vi "Test11ACiR.vi"(8 "errin":errorcluster, 9 "L2T 2":T1 caption="Limites de test pris en compte", 10 "result string":string, 11 "SN":string) -> (0 "error out":errorcluster, 4 "String":string)   [LabVIEW 2020]
uses:
  Ctrl/L2T.ctl
  <vilib>/regexp/Match Regular Expression.xnode
panel:
  # "Pre DCIR_____________________________________"
  # "intra DCIR_____________________________________"
  # "Post DCIR_____________________________________"
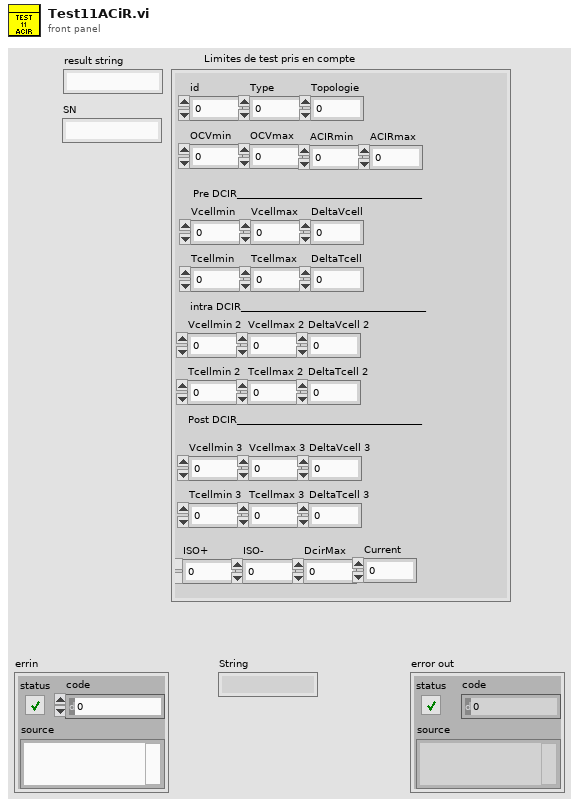
[diagram p1: front panel]
types:
  T1 = typedef "L2T.ctl" = cluster{"id":dbl, "Type":dbl, "OCVmin":dbl, "OCVmax":dbl, "ACIRmin":dbl, "ACIRmax":dbl, "Vcellmin":dbl, "Vcellmax":dbl, "DeltaVcell":dbl, "Tcellmin":dbl, "Tcellmax":dbl, "DeltaTcell":dbl, "ISO+":dbl, "ISO-":dbl, "DcirMax":dbl, "Current":dbl, "Topologie":dbl, "Vcellmin 2":dbl, "Vcellmax 2":dbl, "DeltaVcell 2":dbl, "Tcellmin 2":dbl, "Tcellmax 2":dbl, "DeltaTcell 2":dbl, "Vcellmin 3":dbl, "Vcellmax 3":dbl, "DeltaVcell 3":dbl, "Tcellmin 3":dbl, "Tcellmax 3":dbl, "DeltaTcell 3":dbl}
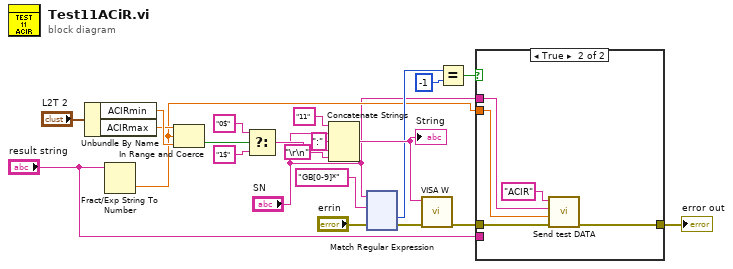
[diagram p0: block diagram]
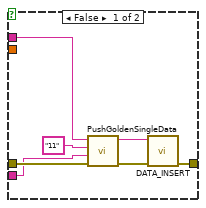
[diagram p2: hidden frame]
diagram:
  n1 = Unbundle By Name("L2T 2") -> ("ACIRmin"=w19:dbl, "ACIRmax"=w18:dbl)
  n2 = Fract/Exp String To Number(string="result string") -> (number=w5:dbl)  [unwired: 3 in, 1 out]
  n3 = In Range and Coerce(upper limit=w18, x=w5, lower limit=w19) -> (In Range?=w20:bool)  [unwired: 1 out]
  n4 = Select(t="0$" ("chaîne"), s=w20, f="1$" ("chaîne")) -> (s? t:f=w17:string)
  n5 = Concatenate Strings("11" ("chaîne"), "SN", ":" ("string"), w17, "\r\n") -> (w22:string)
  "String" <- w22
  n6 = xnode "Match Regular Expression"("input string"="SN", "regular expression"="GB[0-9]*", "error in"="errin") -> ("offset past match"=w11:i32, "error out"=w8:errorcluster)  [unwired: 3 in, 3 out]
  n7 = call "VISA W.vi"("errin"=w8, "Chaîne"=w22) -> ("errout"=w6:errorcluster)  [unwired: 9 in]
  n8 = Equal?(x=w11, y=-1) -> (x = y?=w7:bool)
  n9 = case shown="True" w7 {
    tunnel: w6 -> [w28 w34]
    tunnel: w5 -> [_ w33]
    tunnel: "SN" -> [w27 w32]
    tunnel: [w24 w30] -> w3
    tunnel: "result string" -> [w26 _]
    frame False {
      n10 = call "PushGoldenSingleData.vi"("errin"=w28, "Value"=w26, "TestNum"="11", "SN"=w27) -> ("errout"=w25:errorcluster, "String out"=w23:string)  [unwired: 6 in]
      n11 = call <userlib>:"DATA_INSERT.vi"("errin"=w25, "INSERT"=w23) -> ("errout"=w24:errorcluster)  [unwired: 9 in]
    }
    frame True {
      n12 = call "Send test DATA.vi"("errin"=w34, "Value"=w33, "SN"=w32, "test"="ACIR") -> ("error out"=w30:errorcluster)  [unwired: 7 in]
    }
  }
  "error out" <- w3
